vi "Global_SM Write_Data Out.vi"() -> ()   [LabVIEW 2017, in "Wing.lvlib"]
uses:
  Wing.lvlib
panel:
  in  "Wing_SM_Int":i32
  in  "Wing_SM_Bool":bool
  in  "Wing_SM_DBL":dbl
  # "The Names of the Data items in the Global Variable MUST describe who the Single Writer is\nNaming Convention of all Data Items is:   \nLib Name_Loop Name (SM or SEN or ACT)_Data Name\nExamples:\nDrive_ACT_X axis\nGameController_SEN_JoystickLeft\nHopper_SM_AgitatorSpeed"
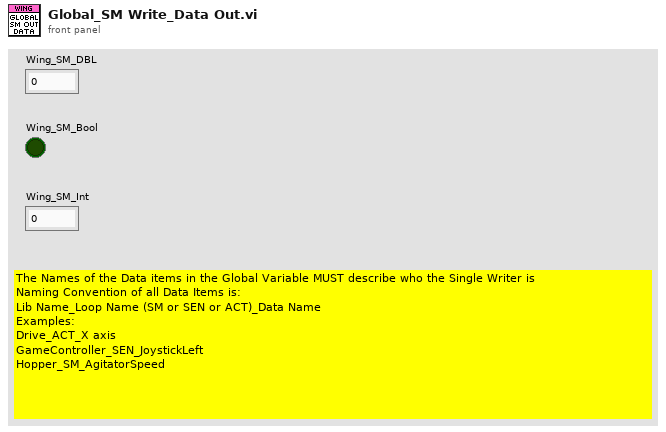
[diagram p1: front panel]
diagram:
